vi "Inc dec thru Function global variable.vi"() -> ()   [LabVIEW 2012]
panel:
  out "Numeric 2":dbl
  in  "Enum":T1(ring)
  in  "Numeric":dbl
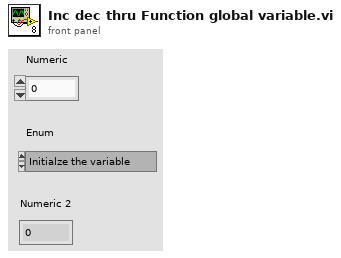
[diagram p1: front panel]
types:
  T1 = enum16{"Initialze the variable", "Increment", "Decrement"}
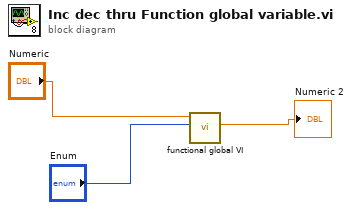
[diagram p0: block diagram]
diagram:
  n1 = call "functional global VI.vi"("Enum"="Enum", "Numeric"="Numeric") -> ("Numeric 2"=→"Numeric 2":dbl)  [unwired: 9 in]
